vi "PicoScope5000aNearestSampleInterval.vi"(5 "Enabled array":i16[](array[numeric])=[0, 0, 0, 0, 0, 0, 0, 0, 0, 0], 6 "Acquisition Settings":T1 {"postTriggerSamples" format="%_6p"; "preTriggerSamples" format="%_6p"}, 8 "error in (no error)":errorcluster, 9 "roundFaster":bool, 10 "timeIntervalRequested":dbl format="%#6_6p", 11 "handle in":i16) -> (0 "error out":errorcluster, 1 "timebase":u32, 2 "timeIntervalAvailable":dbl format="%#6_6p", 3 "handle out":i16)   [LabVIEW 2010]
doc: "Calls Gettimebase function"
uses:
  ps5000a.dll
  shared/Acquisition Settings.ctl
panel:
  in  "Memory Segment":u32
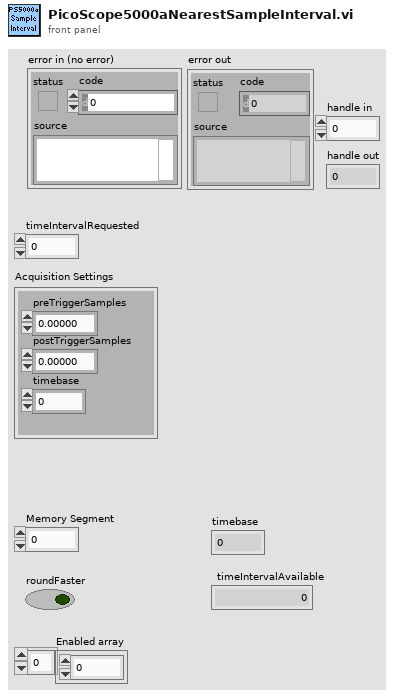
[diagram p1: front panel]
types:
  T1 = typedef "Acquisition Settings.ctl" = cluster{"preTriggerSamples":u64, "postTriggerSamples":u64, "timebase":u32}
  T2 = cluster{"status":bool, "code":u32, "source":string}
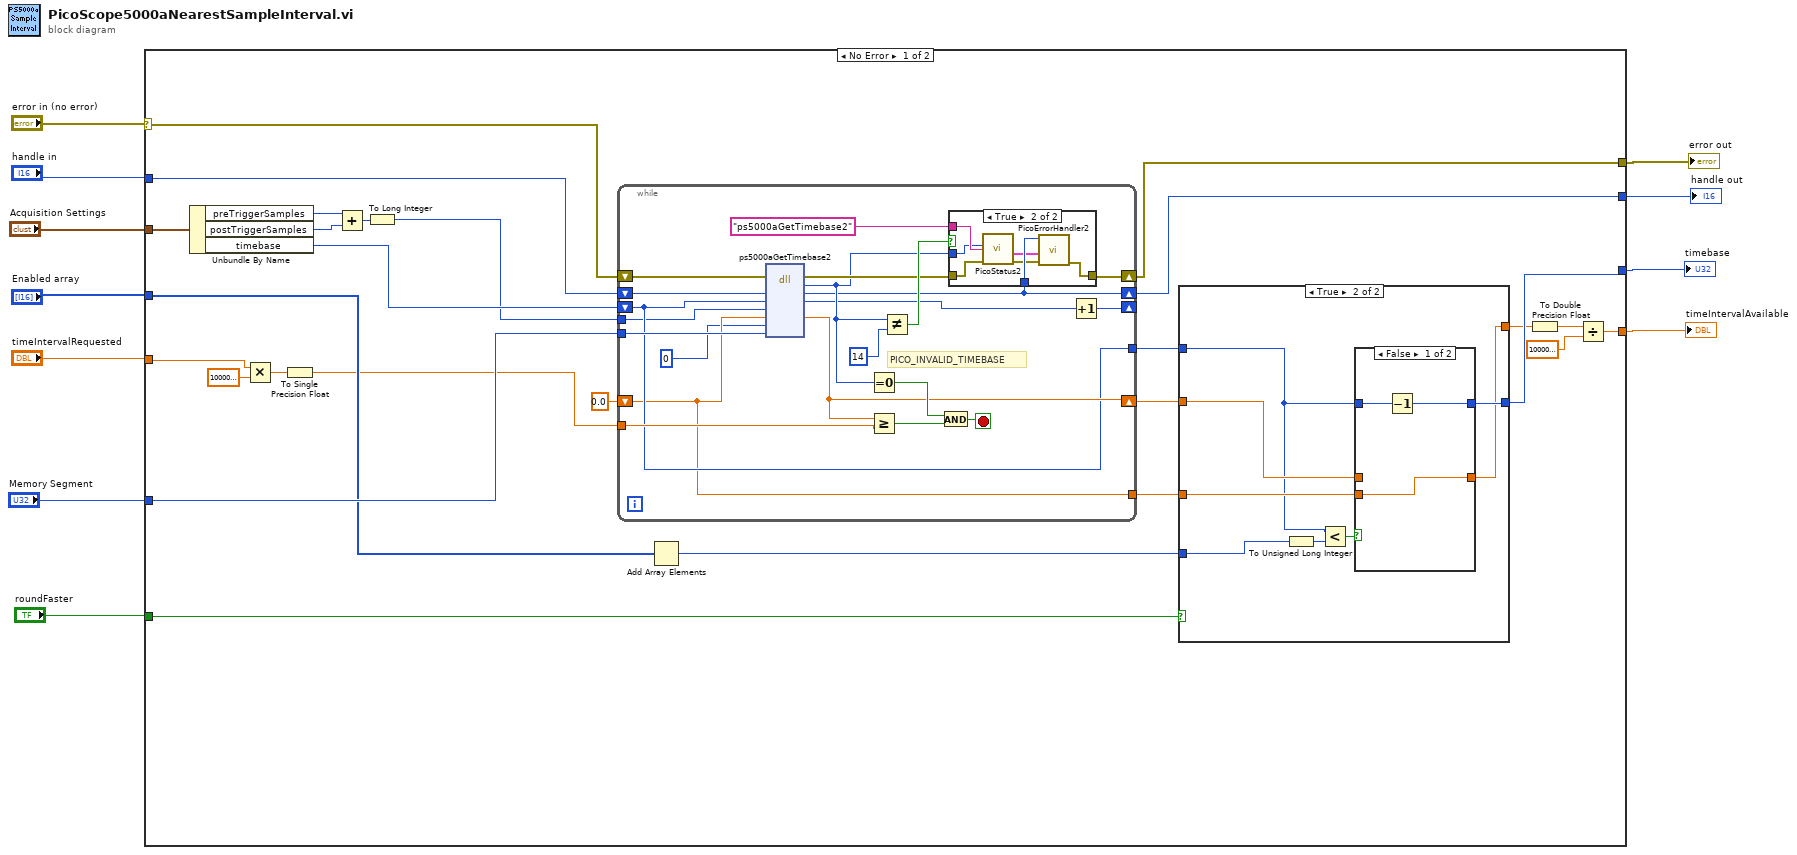
[diagram p0: block diagram]
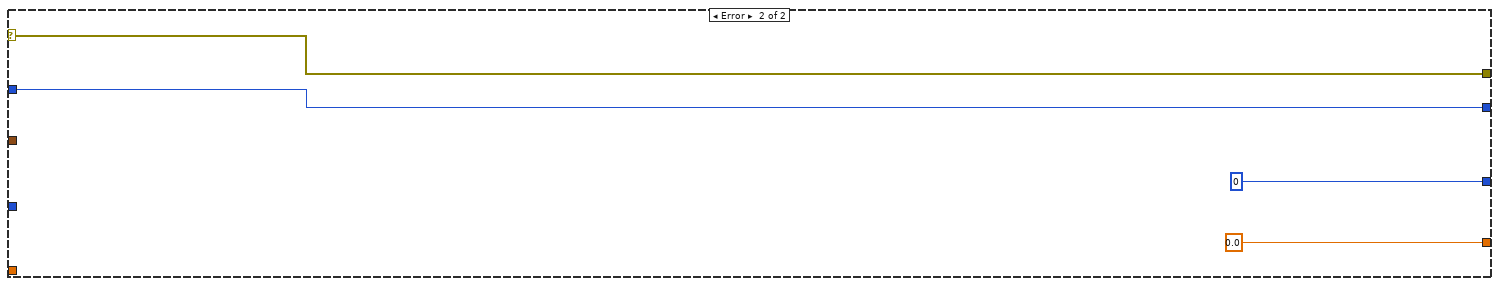
[diagram p5: hidden frame]
diagram:
  n1 = case shown="No Error" "error in (no error)" {
    selector: "error in (no error)" -> [w19 w86]
    tunnel: [w12 w86] -> w11
    tunnel: [w30 w85] -> w10
    tunnel: "handle in" -> [w31 w85]
    tunnel: "Enabled array" -> [w21 _]
    tunnel: "roundFaster" -> [w25 _]
    tunnel: "timeIntervalRequested" -> [w36 _]
    tunnel: [w22 u32 0 ("timebase")] -> w4
    tunnel: [w27 0.0 ("timeIntervalAvailable")] -> w3
    tunnel: "Acquisition Settings" -> [w32 _]
    tunnel: "Memory Segment" -> [w29 _]
    frame No Error {
      n2 = Unbundle By Name(w32) -> ("preTriggerSamples"=w34:u64, "postTriggerSamples"=w35:u64, "timebase"=w26:u32)
      n3 = Multiply(x=w36, y=1000000000.0) -> (x*y=w37:dbl)
      n4 = To Single Precision Float(number=w37) -> (single precision float=w18:sgl)
      n5 = Add(x=w34, y=w35) -> (x+y=w33:u64)
      n6 = To Long Integer(number=w33) -> (32bit integer=w20:i32)
      n7 = while {
        tunnel: w20 -> [w56]
        tunnel: w29 -> [w60]
        shift-right: [w63] -> w30
        shift-left: w31 -> [w58]
        shift-right: [w74] -> w12
        shift-left: w19 -> [w59]
        shift-right: [w72] -> _
        shift-left: w26 -> [w57]
        tunnel: w18 -> [w71]
        shift-right: [w61] -> w23
        shift-left: sgl 0.0 ("timeIntervalNanoseconds") -> [w55]
        tunnel: [w55] -> w24
        tunnel: [w57] -> w14
        stop <- w70 stop-if-true
        # "PICO_INVALID_TIMEBASE"
        n8 = dll-call lib="ps5000a.dll" fn="ps5000aGetTimebase2"(error in=w59, "handle"=w58, "timebase"=w57, "noSamples"=w56, "timeIntervalNanoseconds"=w55, "maxSamples"=0, "segmentIndex"=w60) -> (error out=w65:errorcluster, "PICO_STATUS"=w64:u32, "handle"=w63:i16, "timebase"=w62:u32, "timeIntervalNanoseconds"=w61:sgl)  [unwired: 5 in, 1 out]
        n9 = Equal To 0?(x=w64) -> (x = 0?=w68:bool)
        n10 = Greater Or Equal?(x=w61, y=w71) -> (x >= y?=w69:bool)
        n11 = Not Equal?(x=w64, y=u32 14) -> (x != y?=w66:bool)
        n12 = And(x=w68, y=w69) -> (x .and. y?=w70:bool)
        n13 = case shown="True" w66 {
          tunnel: w65 -> [w75 w82]
          tunnel: [w75 w76] -> w74
          tunnel: "ps5000aGetTimebase2" ("source") -> [_ w81]
          tunnel: w64 -> [_ w80]
          tunnel: w63 -> [_ w79]
          frame False {
          }
          frame True {
            n14 = call "PicoStatus2.vi"("PICO source"=w81, "Error in"=w82, "PICO STATUS"=w80) -> ("error out"=w77:errorcluster, "PICO_STATUS out"=w78:T2)  [unwired: 5 in]
            n15 = call "PicoErrorHandler2.vi"("error in (no error)"=w77, "PICO_STATUS in"=w78, "handle In"=w79) -> ("error out"=w76:errorcluster)  [unwired: 8 in]
          }
        }
        n16 = Increment(x=w62) -> (x+1=w72:u32)
      }
      n17 = Add Array Elements(numeric array=w21) -> (sum=w13:i16)
      n18 = case shown="True" w25 {
        tunnel: [w40 w47] -> w15
        tunnel: w24 -> [_ w46]
        tunnel: w23 -> [w40 w45]
        tunnel: [w39 w48] -> w22
        tunnel: w14 -> [w39 w43]
        tunnel: w13 -> [_ w41]
        frame False {
        }
        frame True {
          n19 = To Unsigned Long Integer(number=w41) -> (unsigned 32bit integer=w42:u32)
          n20 = Less?(x=w43, y=w42) -> (x < y?=w44:bool)
          n21 = case shown="False" w44 {
            tunnel: [w51 w53] -> w48
            tunnel: w43 -> [w50 w53]
            tunnel: [w49 w52] -> w47
            tunnel: w46 -> [w49 _]
            tunnel: w45 -> [_ w52]
            frame False {
              n22 = Decrement(x=w50) -> (x-1=w51:u32)
            }
            frame True {
            }
          }
        }
      }
      n23 = To Double Precision Float(number=w15) -> (double precision float=w16:dbl)
      n24 = Divide(x=w16, y=1000000000.0) -> (x/y=w27:dbl)
    }
    frame Error {
    }
  }
  "error out" <- w11
  "handle out" <- w10
  "timebase" <- w4
  "timeIntervalAvailable" <- w3
